vi "Sort 1D String Array.vi"(4 "1D String[]":string[](array[string])) -> (0 "Sorted Index[]":i32[](array[numeric]), 1 "Sorted 1D String[]":string[](array[string]))   [LabVIEW 2016, in "SLL String.lvlib"]
doc: "Alpha Numeric Sorting of 1D String Array so that strings are ordered like File 1, File 2..File 10 instead of the usual sorting like File 1, File 10, File 2.."
uses:
  SLL String.lvlib
  _Typedefs/Sortable Alpha Numeric Cluster.ctl
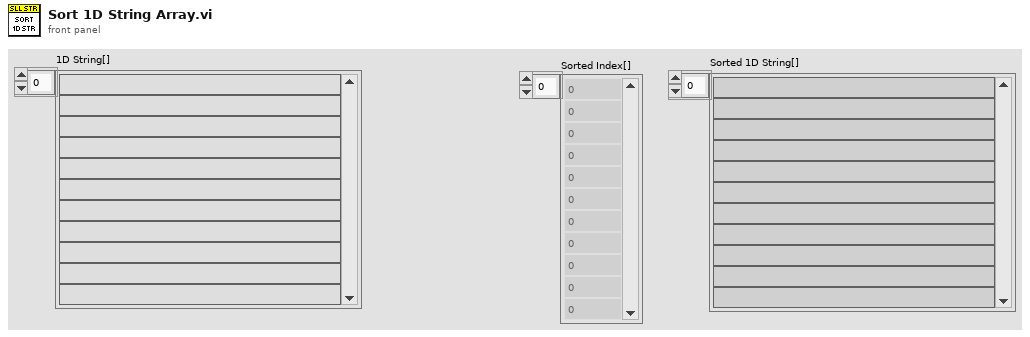
[diagram p1: front panel]
types:
  T1 = typedef "SLL String.lvlib/Sortable Alpha Numeric Cluster.ctl" = cluster{"Numeric[]":dbl[], "String":string}
  T2 = cluster{"Sortable Cluster[]":T1[], "Input String":string, "Index":i32}
  T3 = cluster{"Sortable Cluster[]":T1[], "Input String":string, "Index":i32}[]
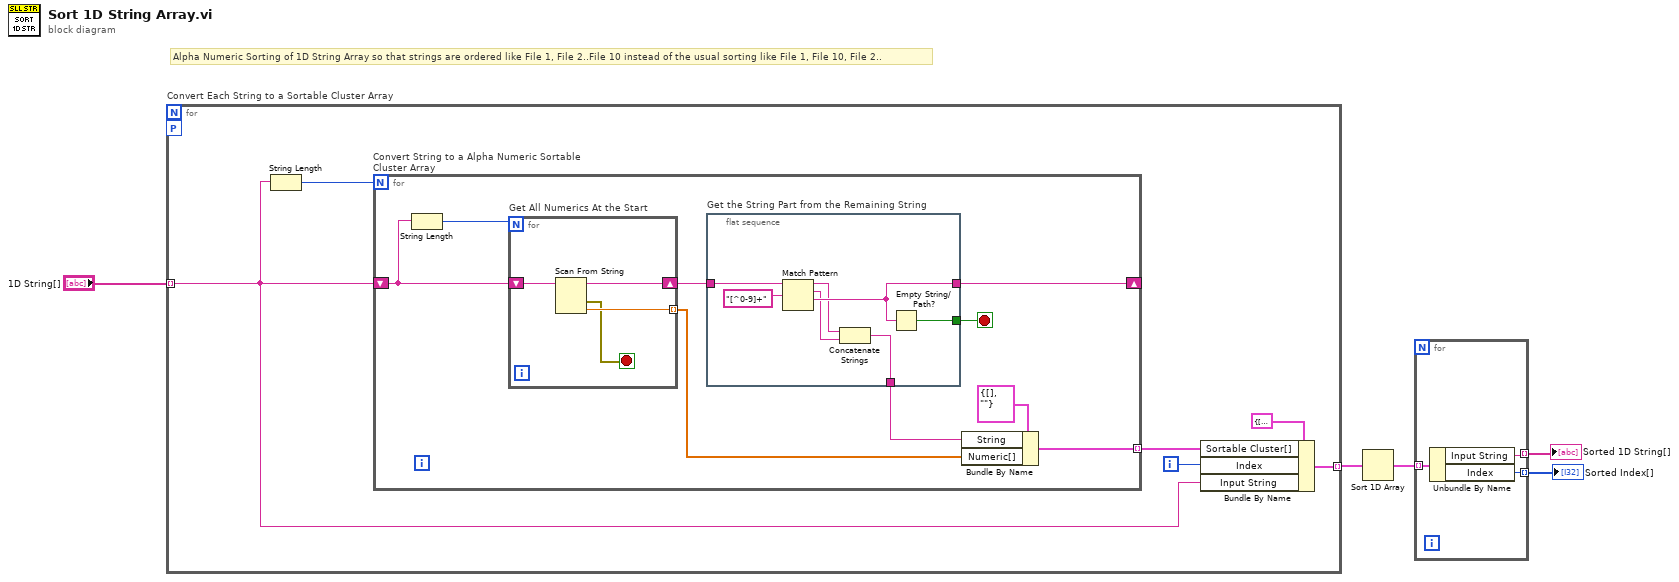
[diagram p0: block diagram]
diagram:
  # "Alpha Numeric Sorting of 1D String Array so that strings are ordered like File 1, File 2..File 10 instead of the usual sorting like File 1, File 10, File 2.."
  n1 = for "Convert Each String to a Sortable Cluster Array" {
    tunnel: "1D String[]" -> [w6] mode=indexing
    workers-P: _ -> [_]
    tunnel: [w7] -> w4 mode=indexing
    i -> [w8]
    n2 = String Length(string=w6) -> (length=w11:i32)
    n3 = for "Convert String to a Alpha Numeric Sortable Cluster Array" {
      N: w11 -> [_]
      shift-right: [w14] -> _
      shift-left: w6 -> [w16]
      tunnel: [w17] -> w9 mode=indexing
      stop <- w13 stop-if-true
      n4 = String Length(string=w16) -> (length=w15:i32)
      n5 = for "Get All Numerics At the Start" {
        N: w15 -> [_]
        shift-right: [w30] -> w20
        shift-left: w16 -> [w31]
        tunnel: [w29] -> w18 mode=indexing
        stop <- w28 stop-if-true
        n6 = Scan From String(input string=w31) -> (remaining string=w30:string, error out=w28:errorcluster, output 1=w29:dbl)  [unwired: 4 in, 1 out]
      }
      n7 = flat-sequence "Get the String Part from the Remaining String" {
        tunnel: w20 -> [w26]
        tunnel: [w24] -> w14
        tunnel: [w27] -> w13
        tunnel: [w21] -> w12
        frame #0 {
          n8 = Match Pattern(string=w26, regular expression="[^0-9]+" ("format string")) -> (before substring=w23:string, match substring=w22:string, after substring=w24:string)  [unwired: 1 in, 1 out]
          n9 = Concatenate Strings(w23, w22) -> (w21:string)
          n10 = Empty String/Path?(string/path=w24) -> (empty?=w27:bool)
        }
      }
      n11 = Bundle By Name(cluster=T1 {"Numeric[]"=[], "String"=""}, "String"=w12, "Numeric[]"=w18) -> (w17:T1)
    }
    n12 = Bundle By Name(cluster=T2 {"Sortable Cluster[]"=[], "Input String"="", "Index"=0}, "Sortable Cluster[]"=w9, "Index"=w8, "Input String"=w6) -> (w7:T2)
  }
  n13 = Sort 1D Array(array=w4) -> (sorted array=w3:T3)
  n14 = for {
    tunnel: w3 -> [w34] mode=indexing
    tunnel: [w33] -> w2 mode=indexing
    tunnel: [w32] -> w1 mode=indexing
    n15 = Unbundle By Name(w34) -> ("Input String"=w33:string, "Index"=w32:i32)
  }
  "Sorted 1D String[]" <- w2
  "Sorted Index[]" <- w1
